vi "TEST - LZW CompressDecompress.vi"(8 "error in (no error)":errorcluster) -> (0 "error out":errorcluster, 2 "pass":bool)   [LabVIEW 2020]
uses:
  <userlib>/_OpenG.lib/error/error.llb/openg_error.lvlib
panel:
  out "Array":i32[](array[numeric])
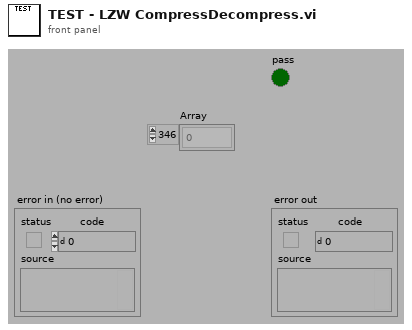
[diagram p1: front panel]
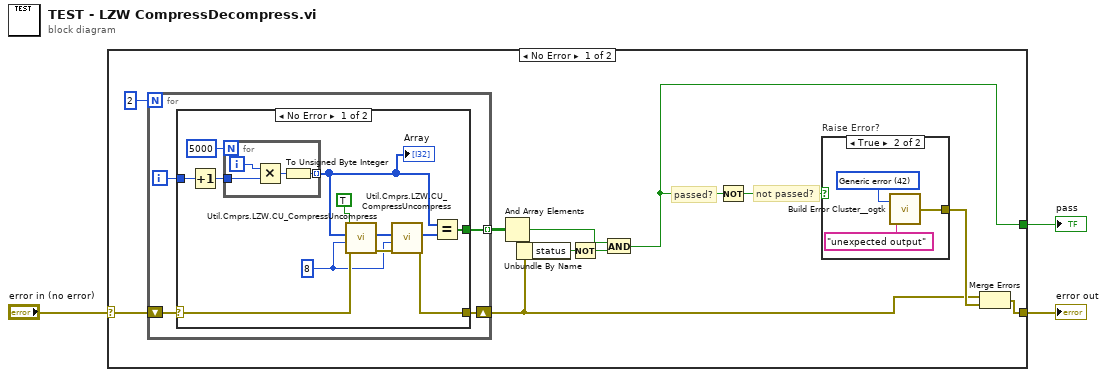
[diagram p0: block diagram]
diagram:
  n1 = case shown="No Error" "error in (no error)" {
    selector: "error in (no error)" -> [w10 w39]
    tunnel: [w7 _] -> w3
    tunnel: [w14 w39] -> w1
    frame No Error {
      # "not passed?"
      # "passed?"
      n2 = for {
        N: 2 -> [_]
        shift-right: [w15] -> w5
        shift-left: w10 -> [w16]
        tunnel: [w17] -> w4 mode=indexing
        i -> [w18]
        n3 = case shown="No Error" w16 {
          selector: w16 -> [w22 w35]
          tunnel: w18 -> [w29 _]
          tunnel: [w23 _] -> w17
          tunnel: [w21 w35] -> w15
          frame No Error {
            w19 = 8 ("LZWBits")
            n4 = Increment(x=w29) -> (x+1=w28:i32)
            n5 = for {
              N: 5000 -> [_]
              tunnel: w28 -> [w34]
              tunnel: [w31] -> w20 mode=indexing
              i -> [w33]
              n6 = Multiply(x=w33, y=w34) -> (x*y=w32:i32)
              n7 = To Unsigned Byte Integer(number=w32) -> (unsigned 8bit integer=w31:u8)
            }
            "Array" <- w20
            n8 = call "Util.Cmprs.LZW.CU_CompressUncompress.vi"("error in (no error)"=w22, "LZWBits"=w19, "Data"=w20, "Compress/Decompress (T/F)"=TRUE) -> ("error out"=w26:errorcluster, "Data out"=w25:u8[])  [unwired: 6 in]
            n9 = call "Util.Cmprs.LZW.CU_CompressUncompress.vi"("error in (no error)"=w26, "LZWBits"=w19, "Data"=w25) -> ("error out"=w21:errorcluster, "Data out"=w27:u8[])  [unwired: 7 in]
            n10 = Equal?(x=w20, y=w27) -> (x = y?=w23:bool[])
          }
          frame Error {
          }
        }
      }
      n11 = And Array Elements(Boolean array=w4) -> (logical AND=w8:bool)
      n12 = Unbundle By Name(w5) -> ("status"=w11:bool)
      n13 = Not(x=w11) -> (.not. x?=w9:bool)
      n14 = And(x=w8, y=w9) -> (x .and. y?=w7:bool)
      n15 = Not(x=w7) -> (.not. x?=w12:bool)
      n16 = case "Raise Error?" shown="True" w12 {
        tunnel: [_ w36] -> w13
        frame False {
        }
        frame True {
          w37 = 42 items=["No error", "Argument error", "Memory is full", "Out of zone", "End of file", "File already open", "Generic file I/O error", "File not found", "File permission error", "Disk is full", "Duplicate path", "Too many files open", "System feature not enabled", "Resource file not found", "Cannot add resource", "Resource not found", "Image not found", "Image memory error", "Pen does not exist", "Config type invalid", "Config token not found", "Config parse error", "Config memory error", "Bad external code format", "Bad external code offset", "External code not present", "Null window", "Destroy window error", "Null menu", "Print aborted", "Bad print record", "Print driver error", "Windows error during printing", "Memory error during printing", "Print dialog error", "Generic print error", "Invalid device refnum", "Device not found", "Device parameter error", "Device unit error", "Cannot open device", "Device call aborted", "Generic error", "Cancelled by user", "Object ID too low", "Object ID too high", "Object not in heap", "Unknown heap", "Unknown object (invalid DefProc)", "Unknown object (DefProc not in table)", "Message out of range", "Invalid (null) method", "Unknown message", "Manager call not supported", "Bad address", "Network operation in progress", "Network operation timed out", "Connection is busy", "Network attribute not supported", "Network error", "Address in use", "System out of memory", "Connection aborted", "Connection refused", "Not connected", "Already connected", "Connection closed", "Initialization error (interapplication manager)", "Bad occurrence", "Wait on unbound occurrence handler", "Occurrence queue overflow", "Datalog type conflict", "Unused", "Unrecognized type (interapplication manager)", "Memory corrupt", "Failed to make temporary DLL", "Old CIN version", "Drag socket not found", "Failed to load drop-object", "Failed to register OLE object", "Failed to release OLE object", "Format specifier type mismatch", "Unknown format specifier", "Too few format specifiers", "Too many format specifiers", "Scan failed", "Newer CIN version", "Error converting to variant", "Runtime menu error", "Password tampered", "Variant attribute not found", "Incompatible variant data type", "Event data is not available", "Event Store is not present", "Occurrence is not found", "Event Queue is not created", "Event info is not available", "Refnum passed is NULL", "Error retrieving Class GUID", "Error retrieving CoClass GUID", "Error retrieving TypeLib GUID.", "Bad built application magic bytes.", "Specific driver is different from the specific driver associated with the Logical Name.", "There is no session opened to the class driver.", "Max Error", "MAX - Error with config objects", "MAX - Error loading configuration", "MAX - Group not supported"]
          n17 = call <userlib>:"Build Error Cluster__ogtk.vi"("String to Prepend to source (\"\")"="unexpected output" ("String to Prepend to source (\"\")"), "code"=w37) -> ("error out"=w36:errorcluster)
        }
      }
      n18 = Merge Errors(w5, w13) -> (w14:errorcluster)
    }
    frame Error {
    }
  }
  "pass" <- w3
  "error out" <- w1
